vi "uA_daq_Set_ext_power_CM2_DIANA_LOG_Bat.vi"(11 "USB DAQ in":tag) -> (0 "error out":errorcluster, 3 "USB DAQ out":tag)   [LabVIEW 2015]
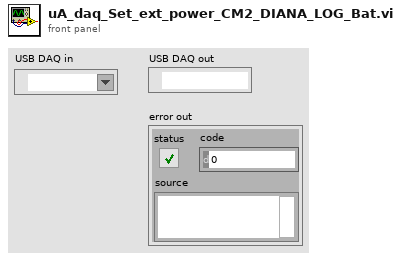
[diagram p1: front panel]
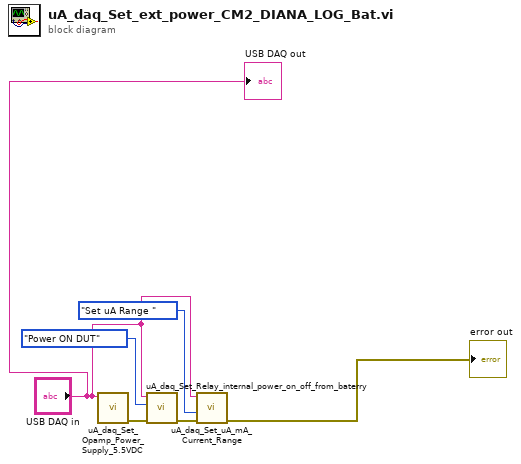
[diagram p0: block diagram]
diagram:
  n1 = call "uA_daq_Set_Opamp_Power_Supply_5.5VDC.vi"("USB DAQ"="USB DAQ in") -> ("error out"=w2:errorcluster)  [unwired: 10 in]
  n2 = call "uA_daq_Set_Relay_internal_power_on_off_from_baterry.vi"("error in"=w2, "Power ON/OFF DUT"=enum16{"Power ON DUT", "Power OFF DUT"}."Power ON DUT", "USB DAQ"="USB DAQ in") -> ("error out"=w4:errorcluster)  [unwired: 8 in]
  n3 = call "uA_daq_Set_uA_mA_Current_Range.vi"("error in"=w4, "Current Range"=enum16{"Set uA Range ", "Set mA Range"}."Set uA Range ", "device name"="USB DAQ in") -> ("error out"=→"error out":errorcluster)  [unwired: 8 in]
  "USB DAQ out" <- "USB DAQ in"
